vi "Test Flatten.vi"() -> ()   [LabVIEW 2021]
uses:
  FIFO_DAQ/CIF_NIChn_FIFO_DAQ.lvclass
  CIFChannels/Typedef/Direction.ctl
  CIFChannels/CIFChannels.lvclass
  ChannelCommon/typedef/FIFO Header.ctl
  ChannelCommon/ChannelCommon.lvlib
  ChannelCommon/typedef/Datatype Waveform.ctl
  ChannelCommon/typedef/TimeStamps.ctl
panel:
  in  "FIFO Timestamps":T1={"ClockID"=2, "T0"=432, "T_Out"=543}
  out "Data out":T2[](array[typedef])=[{"measurement"=[0.0, 0.0, 0.0, 0.0, 0.0, 0.0, 0.0, 3.14], "dT"=0.01, "Timestamp"=498, "Read Lock"=FALSE}, {"measurement"=[0.0, 0.0, 0.0, 0.0, 0.0, 0.0, 0.0, 9.8], "dT"=0.12, "Timestamp"=12345, "Read Lock"=FALSE}]
  in  "Data In":T2[](array[typedef])=[{"measurement"=[0.0, 0.0, 0.0, 0.0, 0.0, 0.0, 0.0, 3.14], "dT"=0.01, "Timestamp"=498, "Read Lock"=FALSE}, {"measurement"=[0.0, 0.0, 0.0, 0.0, 0.0, 0.0, 0.0, 9.8], "dT"=0.12, "Timestamp"=12345, "Read Lock"=FALSE}]
  out "Header":T3={"Length"=57, "T0"=432, "T_Out"=543, "T_Tx"=1727639110950812000, "Ctr"=1, "ClockID"=2}
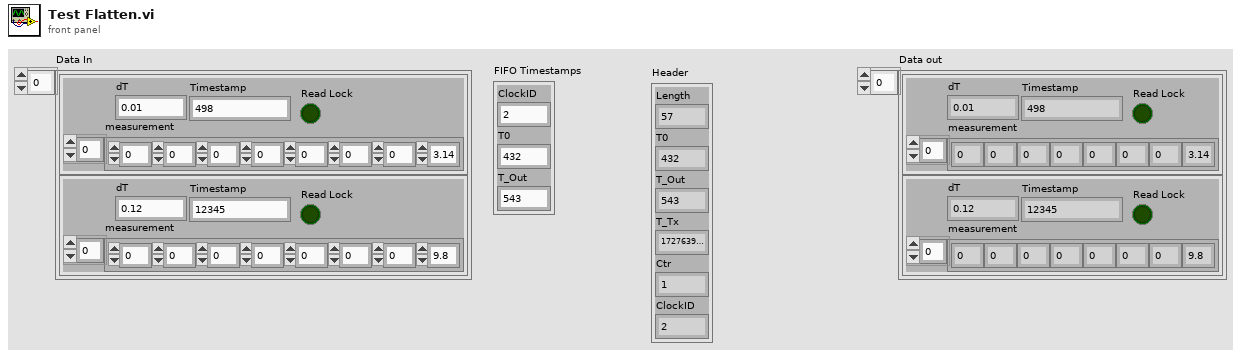
[diagram p1: front panel]
types:
  T1 = typedef "ChannelCommon.lvlib/TimeStamps.ctl" = cluster{"ClockID":u8, "T0":i64, "T_Out":i64}
  T2 = typedef "ChannelCommon.lvlib/Datatype Waveform.ctl" = cluster{"measurement":dbl[], "dT":dbl, "Timestamp":i64, "Read Lock":bool}
  T3 = typedef "ChannelCommon.lvlib/FIFO Header.ctl" = cluster{"Length":u64, "T0":i64, "T_Out":i64, "T_Tx":i64, "Ctr":u64, "ClockID":u8}
  T4 = typedef "CIFChannels.lvclass/Direction.ctl" = enum16{"Publisher", "Subscriber"}
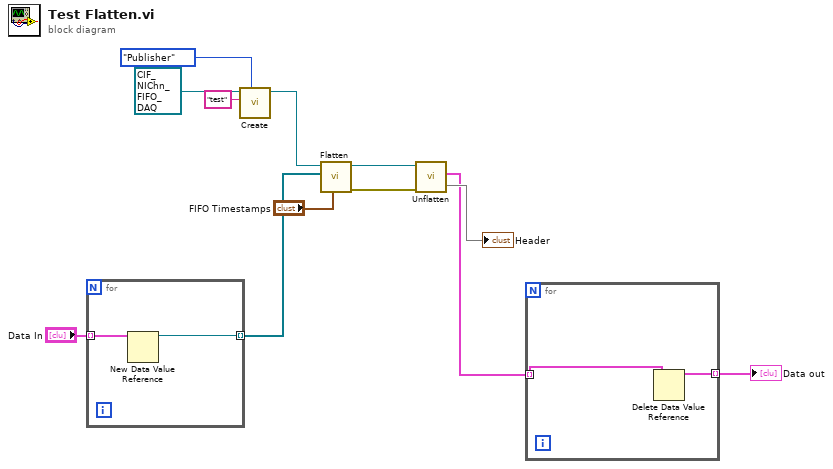
[diagram p0: block diagram]
diagram:
  n1 = for {
    tunnel: "Data In" -> [w14] mode=indexing
    tunnel: [w13] -> w7 mode=indexing
    n2 = New Data Value Reference(data value=w14) -> (data value reference=w13:refnum<data-value>)  [unwired: 1 in, 1 out]
  }
  n3 = call-dynamic "Create.vi"("Direction"=Direction."Publisher", "Name"="test", "CIFFIFO in"=refnum<class "CIF_NIChn_FIFO_DAQ.lvclass"> refnum ("CIF_NIChn_Fifo_Power.lvclass")) -> ("CIFFIFO out"=w4:refnum<class "CIF_NIChn_FIFO_DAQ.lvclass">)  [unwired: 7 in, 1 out]
  n4 = call "Flatten.vi"("FIFO Timestamps"="FIFO Timestamps", "Data In"=w7, "CIF_NIChn_FIFO_DAQ in"=w4) -> ("error out"=w11:errorcluster, "CIF_NIChn_FIFO_DAQ out"=w12:refnum<class "CIF_NIChn_FIFO_DAQ.lvclass">)  [unwired: 6 in, 1 out]
  n5 = call "Unflatten.vi"("error in (no error)"=w11, "CIF_NIChn_FIFO_DAQ in"=w12) -> ("DAQ Out"=w6:T2[], 4:→"Header")  [unwired: 5 in, 3 out]
  n6 = for {
    tunnel: w6 -> [w15] mode=indexing
    tunnel: [w16] -> w5 mode=indexing
    n7 = Delete Data Value Reference(data value reference=w15) -> (data value=w16:T2)  [unwired: 1 in, 1 out]
  }
  "Data out" <- w5
